vi "Data_get_joe_3.3.vi"() -> ()   [LabVIEW 2011]
uses:
  <vilib>/Utility/error.llb/DialogType.ctl
  <vilib>/Analysis/2dsp.llb/Real FFT.vi
  <vilib>/Analysis/NI_AALPro.lvlib
panel:
  out "Tab Control":T1(tab)
  in  "freq. step (GHz)":dbl=0.0003 min=0.00025 max=67.0 step=1e-06 format="%#.12f"
  in  "number of steps":u32=1 min=1 step=1
  in  "Filter up to (MHz)":ext=2.5
  in  "Chirp start (MHz)":ext=2.5
  in  "Channel Number":u16=1
  in  "Amount of averagings":u32=10 min=1 step=1
  out "Busy":bool
  out "#points":u32
  out "read time (ms)":u32
  in  "time/div":T2(ring)
  in  "time/point":T3(ring)
  in  "TDS VISA Port":refnum<visa-resource-name>="GPIB0::1::INSTR"
  in  "PSG1 VISA Port":refnum<visa-resource-name>="GPIB0::1::INSTR"
  in  "PSG1 start freq. (GHz)":dbl=0.0003 min=0.00025 max=67.0 step=1e-06 format="%#.12f"
  in  "PSG1 Ampl (dBm)":dbl min=-135.0 max=30.0 step=0.5 format="%#_8g"
  in  "Auto":bool caption="Autosave"
  in  "Automatic Overwrite?":bool
  out "f cur. (GHz)":i32
  in  "File Extension":string="ccd"
  in  "File Name":string="trace"
  in  "Folder":path
  in  "PSG2 Ampl (dBm)":dbl min=-135.0 max=30.0 step=0.5 format="%#_8g"
  in  "PSG2 freq. offset (GHz)":dbl=0.0003 min=0.00025 max=67.0 step=1e-06 format="%#.12f"
  in  "PSG2 VISA Port":refnum<visa-resource-name>="GPIB0::1::INSTR"
  in  "Chirp up to (GHz)":dbl
  in  "#Sweeps":u32=1 min=1 max=1000 step=1
  out "Current sweep":u32=1 min=1 max=1000 step=1
  in  "FFT every#":u32=1 min=1 max=1000 step=1
  in  "Substr":bool
  out "Frequency Domain Signal":cluster{ext[], dbl[]}(graph)
  out "Time Domain Signal":dbl[](graph)
  out "Data":dbl[](array[numeric])
  out "FFT (Im)":dbl[](array[numeric])
  out "FFT (Re)":dbl[](array[numeric])
  out "Final array":ext[][](array[numeric])
  out "size(s)":i32
  out "tdsavges#":i32 caption="tds averaged:"
  out "Oscilloscope Data":dbl[](array[numeric])
  in  "PauseB":bool caption="Pause"
  in  "Start":bool
  in  "Quit":bool
  in  "Stop":bool
  # "General Settings"
  # "OSC Settings"
  # "PSG1 Settings"
  # "PSG2 Settings"
  # "File Storage"
  # "Spectrum data"
  # "Vi Control"
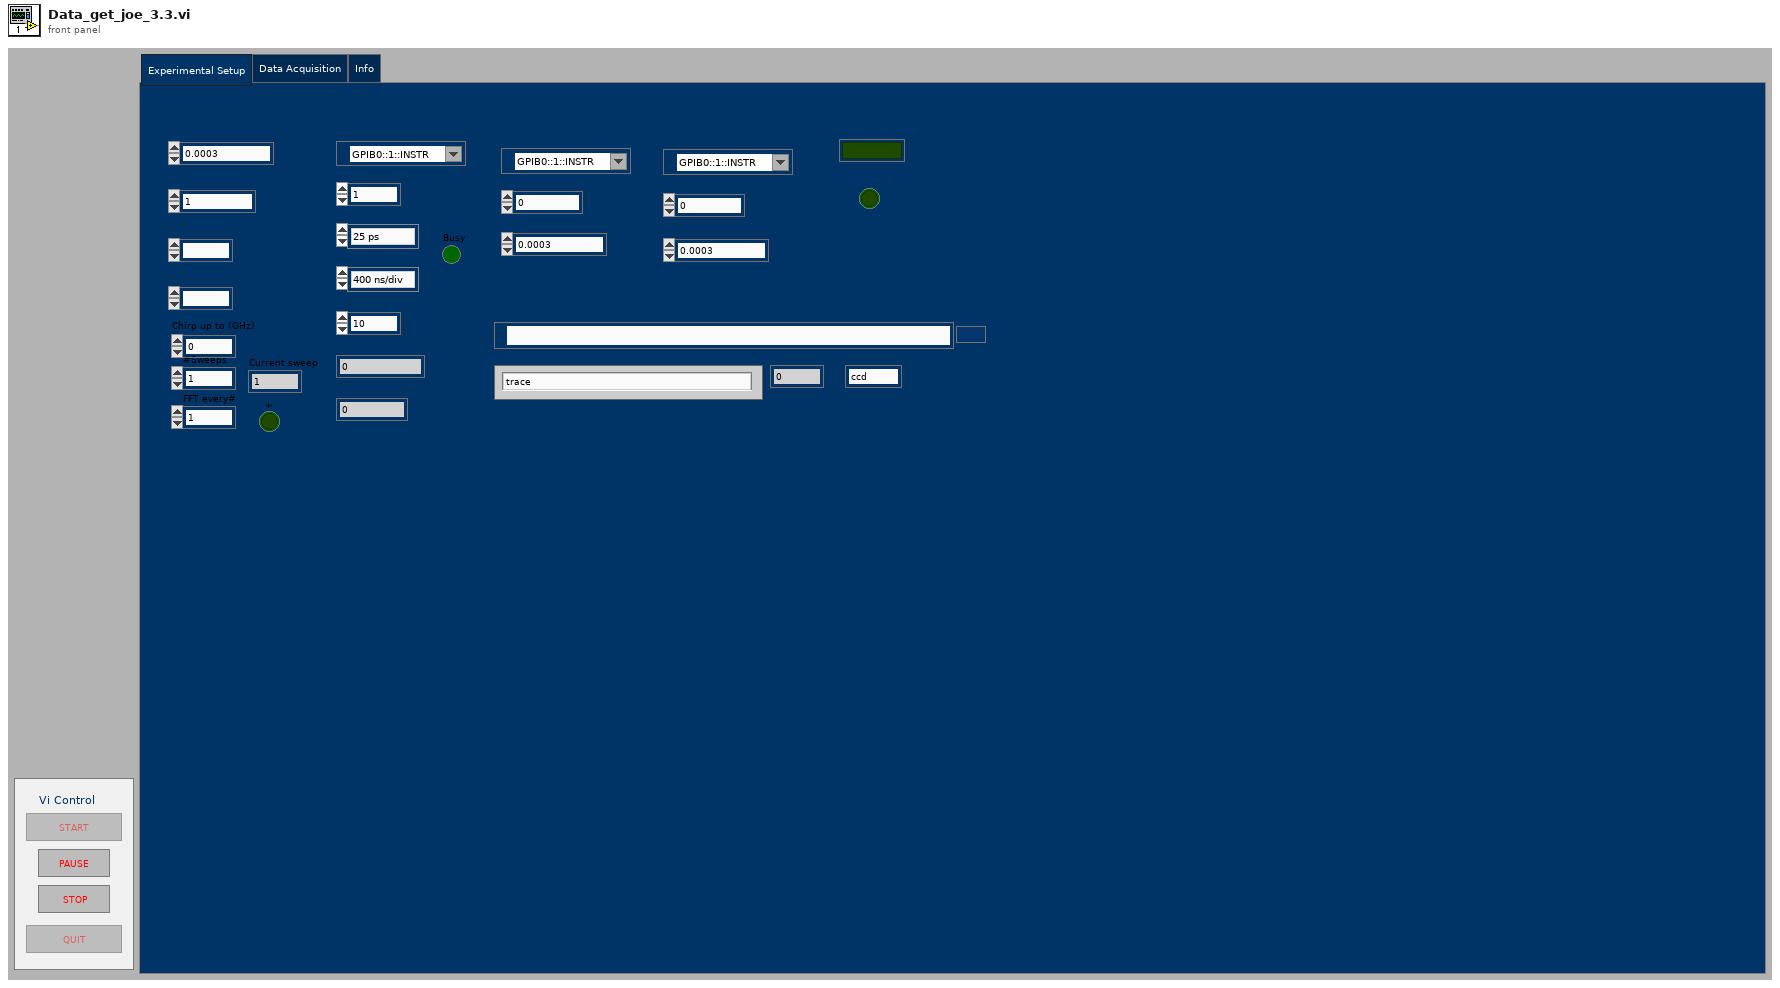
[diagram p1: front panel]
types:
  T1 = enum32{"Experimental Setup", "Data Acquisition", "Info"}
  T2 = enum16{"400 ns/div", "1 us/div", "2 us/div", "4 us/div", "10 us/div", "20 us/div"}
  T3 = enum16{"25 ps", "50 ps", "100 ps", "200 ps", "400 ps", "800 ps", "2 ns"}
  T4 = enum8{"Enabled", "Disabled", "Disabled and Grayed Out"}
  T5 = enum16{"open", "replace", "create", "open or create", "replace or create", "replace or create with confirmation"}
  T6 = typedef "DialogType.ctl" = u16
  T7 = cluster{"Folder":path, "File Name":string, "File Extension":string}
  T8 = cluster{"Folder":path, "Name":string, "Ext":string}
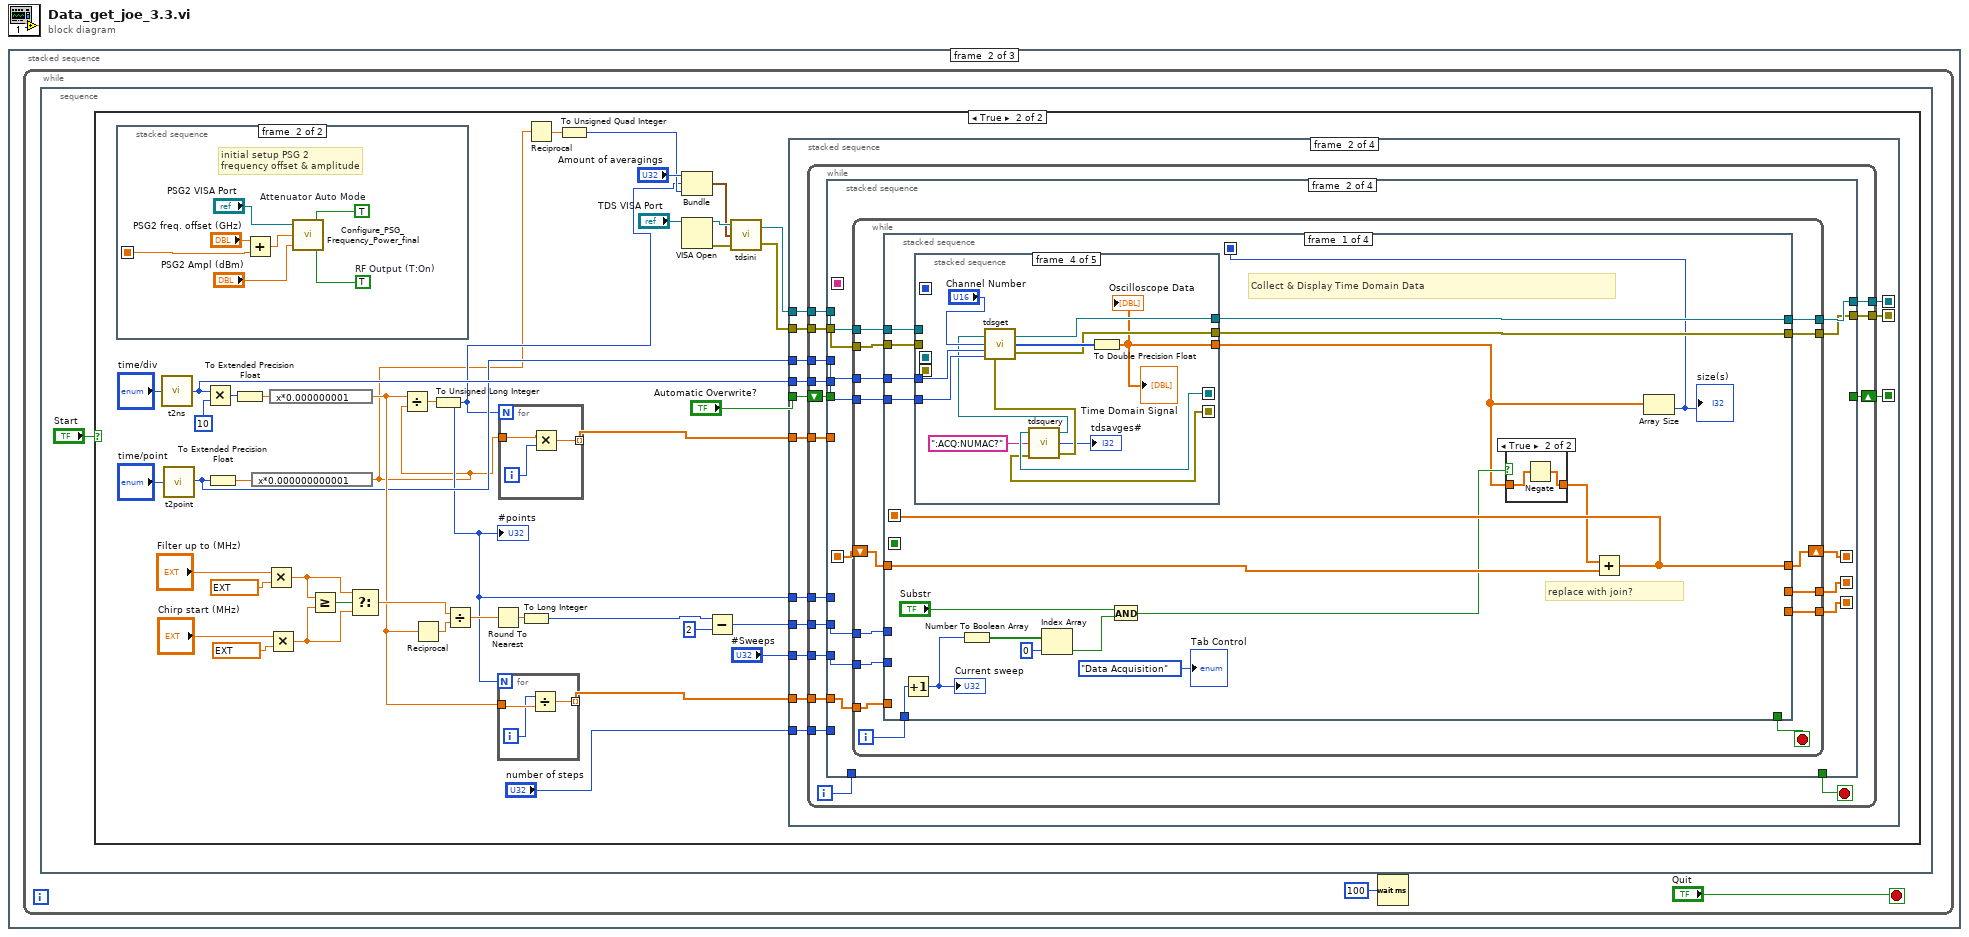
[diagram p0: block diagram]
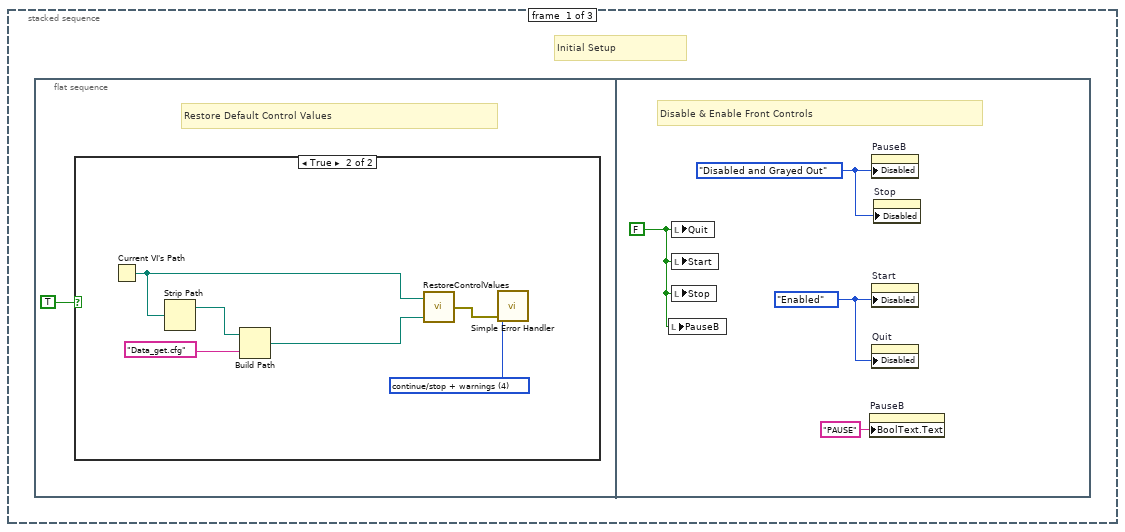
[diagram p2: hidden frame]
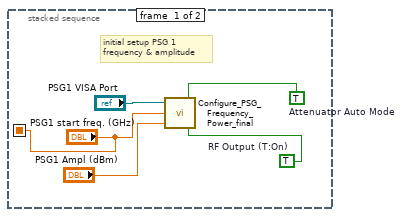
[diagram p5: hidden frame]
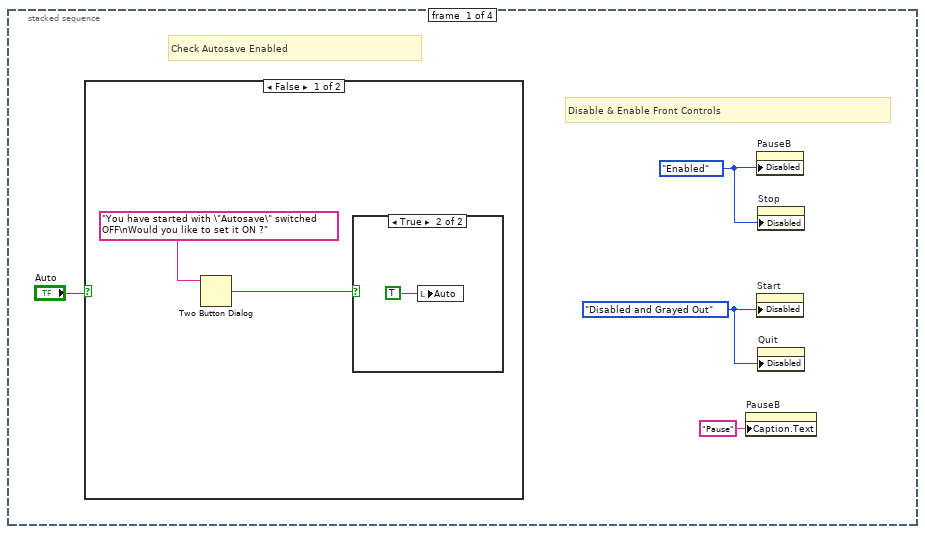
[diagram p6: hidden frame]
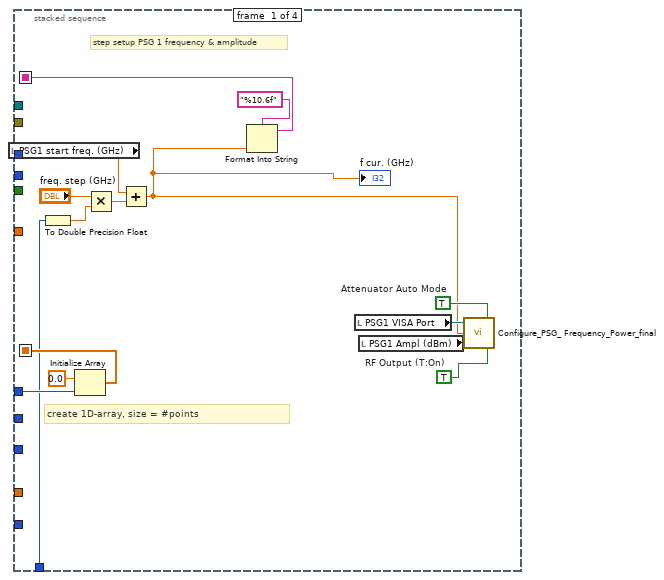
[diagram p9: hidden frame]
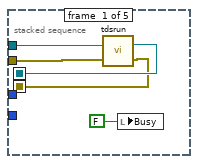
[diagram p11: hidden frame]
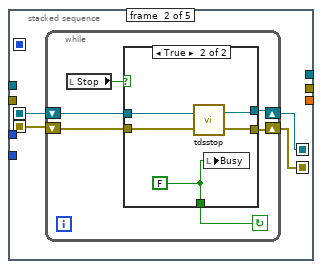
[diagram p12: hidden frame]
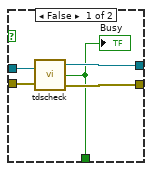
[diagram p13: hidden frame]
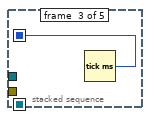
[diagram p14: hidden frame]
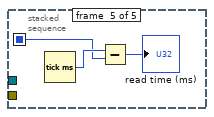
[diagram p15: hidden frame]
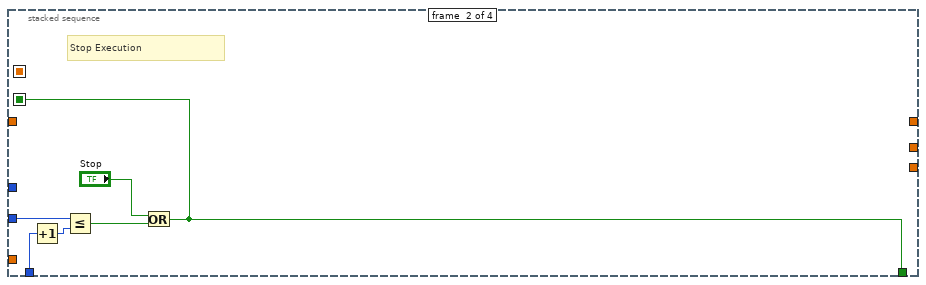
[diagram p16: hidden frame]
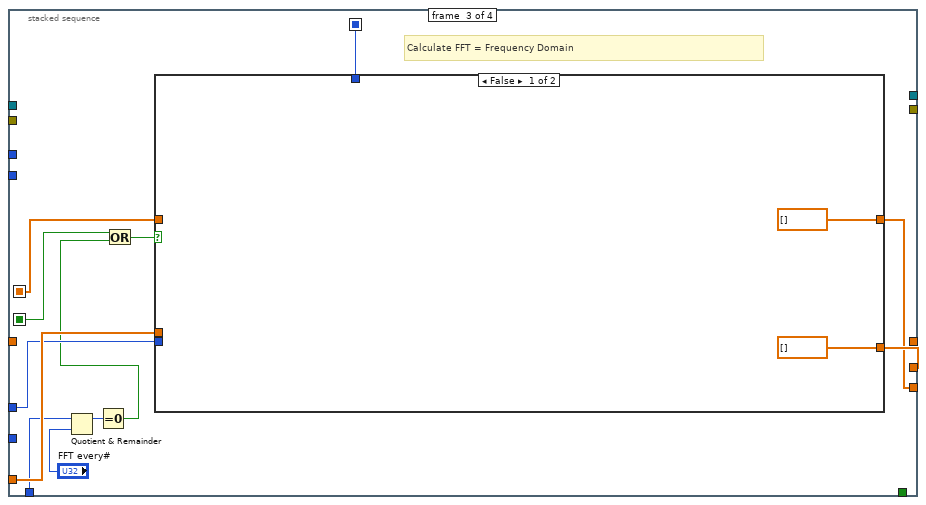
[diagram p17: hidden frame]
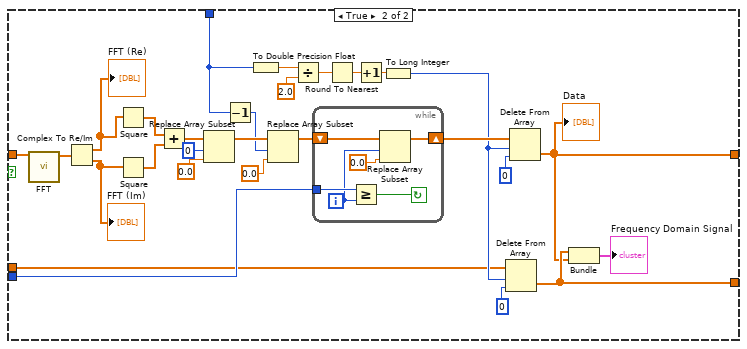
[diagram p18: hidden frame]
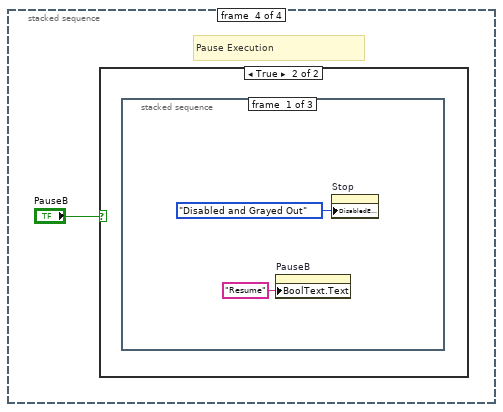
[diagram p19: hidden frame]
diagram:
  n1 = stacked-sequence {
    frame #0 {
      # "Initial Setup"
      n2 = flat-sequence {
        frame #0 {
          # "Restore Default Control Values"
          n3 = case shown="True" TRUE {
            frame False {
            }
            frame True {
              w2 = T6 4 items=["no dialog", "OK message", "continue or stop message", "OK message + warnings", "continue/stop + warnings"] ("type of dialog (OK msg:1)")
              n4 = Current VI's Path() -> (path=w3:path)
              n5 = Strip Path(path=w3) -> (stripped path=w4:path)  [unwired: 1 out]
              n6 = Build Path(base path=w4, name or relative path="Data_get.cfg") -> (appended path=w6:path)
              n7 = call "RestoreControlValues.vi"("file path"=w6, "vi path"=w3) -> ("error out"=w5:errorcluster)
              n8 = call <vilib>:"Simple Error Handler.vi"("type of dialog (OK msg:1)"=w2, "error in (no error)"=w5) -> ()  [unwired: 3 in, 5 out]
            }
          }
        }
        frame #1 {
          w10 = T4."Disabled and Grayed Out" ("Disabled")
          w8 = T4."Enabled" ("Disabled")
          w11 = FALSE ("Quit")
          # "Disable & Enable Front Controls"
          n9 = local write "PauseB"(w11) -> ()
          n10 = local write "Quit"(w11) -> ()
          n11 = local write "Start"(w11) -> ()
          n12 = local write "Stop"(w11) -> ()
          n13 = property on="PauseB" class="Bool (strict)"("BoolText.Text"="PAUSE" ("Boolean Text.Text")) -> ()  [unwired: 2 in, 2 out]
          n14 = property on="PauseB" class="Bool (strict)"("Disabled"=w10) -> ()  [unwired: 2 in, 2 out]
          n15 = property on="Start" class="Bool (strict)"("Disabled"=w8) -> ()  [unwired: 2 in, 2 out]
          n16 = property on="Quit" class="Bool (strict)"("Disabled"=w8) -> ()  [unwired: 2 in, 2 out]
          n17 = property on="Stop" class="Bool (strict)"("Disabled"=w10) -> ()  [unwired: 2 in, 2 out]
        }
      }
    }
    frame #1 {
      n18 = while {
        stop <- "Quit" stop-if-true
        n19 = stacked-sequence {
          frame #0 {
            n20 = case shown="True" "Start" {
              frame False {
              }
              frame True {
                n21 = stacked-sequence {
                  seq-local: ["PSG1 start freq. (GHz)" _] -> [_ w63]
                  frame #0 {
                    w59 = TRUE  # Attenuator Auto Mode
                    w57 = TRUE  # RF Output (T:On)
                    # "initial setup PSG 1 \nfrequency & amplitude"
                    n22 = call "Configure_PSG_ Frequency_Power_final.vi"("RF Output (T:On)"=w57, "Attenuator Auto Mode (T:Enable)"=w59, "Power [dBm]"="PSG1 Ampl (dBm)", "Frequency [GHz]"="PSG1 start freq. (GHz)", "VISA resource name"="PSG1 VISA Port") -> ()
                  }
                  frame #1 {
                    w65 = TRUE  # Attenuator Auto Mode
                    w66 = TRUE  # RF Output (T:On)
                    # "initial setup PSG 2\nfrequency offset & amplitude"
                    n23 = Add(x="PSG2 freq. offset (GHz)", y=w63) -> (x+y=w62:dbl)
                    n24 = call "Configure_PSG_ Frequency_Power_final.vi"("RF Output (T:On)"=w66, "Attenuator Auto Mode (T:Enable)"=w65, "Power [dBm]"="PSG2 Ampl (dBm)", "Frequency [GHz]"=w62, "VISA resource name"="PSG2 VISA Port") -> ()
                  }
                }
                n25 = call "t2ns.vi"("t/div"="time/div") -> ("ns/div"=w27:u32)
                n26 = call "t2point.vi"("t/point"="time/point") -> ("ps/point"=w25:u32)
                n27 = Multiply(x=w27, y=u32 10) -> (x*y=w49:u32)
                n28 = To Extended Precision Float(1:w25) -> (0:w46:ext)
                n29 = To Extended Precision Float(1:w49) -> (0:w47:ext)
                n30 = expression code="x*0.000000000001"(w46) -> (w15:ext)
                n31 = Multiply(x="Filter up to (MHz)", y=ext 1000000.0) -> (x*y=w38:ext)
                n32 = Multiply(x="Chirp start (MHz)", y=ext 1000000.0) -> (x*y=w35:ext)
                n33 = expression code="x*0.000000001"(w47) -> (w29:ext)
                n34 = Greater Or Equal?(x=w38, y=w35) -> (x >= y?=w45:bool)
                n35 = Select(t=w38, s=w45, f=w35) -> (s? t:f=w43:ext)
                n36 = Divide(x=w29, y=w15) -> (x/y=w48:ext)
                n37 = Reciprocal(x=w29) -> (1/x=w44:ext)
                n38 = To Unsigned Long Integer(number=w48) -> (unsigned 32bit integer=w16:u32)
                "#points" <- w16
                n39 = Divide(x=w43, y=w44) -> (x/y=w42:ext)
                n40 = Round To Nearest(number=w42) -> (nearest integer value=w41:ext)
                n41 = for {
                  N: w16 -> [_]
                  tunnel: w29 -> [w463]
                  tunnel: [w464] -> w30 mode=indexing
                  i -> [w462]
                  n42 = Divide(x=w462, y=w463) -> (x/y=w464:ext)
                }
                n43 = for {
                  N: w16 -> [_]
                  tunnel: w15 -> [w467]
                  tunnel: [w466] -> w28 mode=indexing
                  i -> [w465]
                  n44 = Multiply(x=w467, y=w465) -> (x*y=w466:ext)
                }
                n45 = To Long Integer(number=w41) -> (32bit integer=w21:i32)
                n46 = Reciprocal(x=w15) -> (1/x=w31:ext)
                n47 = To Unsigned Quad Integer(1:w31) -> (0:w32:u64)
                n48 = Bundle("Amount of averagings"="Amount of averagings", w16, w32) -> (w33:cluster{"Amount of averagings ":u32, u32, u64})  [unwired: 1 in]
                n49 = VISA Open(VISA resource name="TDS VISA Port") -> (VISA resource name=w51:refnum<visa-resource-name>, error out=w52:errorcluster)  [unwired: 4 in]
                n50 = Subtract(x=w21, y=2) -> (x-y=w19:i32)
                n51 = call "tdsini.vi"("Error In (No Error)"=w52, "Acq_par"=w33, "VISA Port In"=w51) -> ("Error Out"=w53:errorcluster, "VISA Port Out"=w54:refnum<visa-resource-name>)
                n52 = stacked-sequence {
                  seq-local: [_ w80 _ _] -> [_ _ w423 _]
                  seq-local: [_ w79 _ _] -> [_ _ w422 _]
                  seq-local: [_ w74 _ _] -> [_ _ _ w424]
                  tunnel: w54 -> [_ w87 _ _]
                  tunnel: w53 -> [_ w86 _ _]
                  tunnel: w25 -> [_ w85 _ _]
                  tunnel: w27 -> [_ w84 _ _]
                  tunnel: w19 -> [_ w83 _ _]
                  tunnel: w30 -> [_ w82 _ _]
                  tunnel: "#Sweeps" -> [_ w81 _ _]
                  tunnel: w28 -> [_ w76 _ _]
                  tunnel: w16 -> [_ w78 _ _]
                  tunnel: "number of steps" -> [_ w77 _ _]
                  tunnel: "Automatic Overwrite?" -> [_ w75 _ _]
                  frame #0 {
                    w68 = T4."Enabled" ("Disabled")
                    w67 = T4."Disabled and Grayed Out" ("Disabled")
                    # "Check Autosave Enabled"
                    # "Disable & Enable Front Controls"
                    n53 = case shown="False" "Auto" {
                      frame False {
                        n54 = Two Button Dialog(message="You have started with \"Autosave\" switched OFF\nWould you like to set it ON ?") -> (T button?=w71:bool)  [unwired: 2 in]
                        n55 = case shown="True" w71 {
                          frame False {
                          }
                          frame True {
                            n56 = local write "Auto"(TRUE) -> ()
                          }
                        }
                      }
                      frame True {
                      }
                    }
                    n57 = property on="PauseB" class="Bool (strict)"("Caption.Text"="Pause") -> ()  [unwired: 2 in, 2 out]
                    n58 = property on="PauseB" class="Bool (strict)"("Disabled"=w68) -> ()  [unwired: 2 in, 2 out]
                    n59 = property on="Start" class="Bool (strict)"("Disabled"=w67) -> ()  [unwired: 2 in, 2 out]
                    n60 = property on="Stop" class="Bool (strict)"("Disabled"=w68) -> ()  [unwired: 2 in, 2 out]
                    n61 = property on="Quit" class="Bool (strict)"("Disabled"=w67) -> ()  [unwired: 2 in, 2 out]
                  }
                  frame #1 {
                    n62 = while {
                      tunnel: w87 -> [w103]
                      tunnel: w86 -> [w102]
                      tunnel: w85 -> [w101]
                      tunnel: w84 -> [w100]
                      tunnel: w83 -> [w99]
                      tunnel: w82 -> [w98]
                      tunnel: w81 -> [w97]
                      tunnel: [w96] -> w80
                      tunnel: [w95] -> w79
                      tunnel: w78 -> [w94]
                      tunnel: w77 -> [w92]
                      tunnel: w76 -> [w90]
                      shift-right: [w88] -> w74
                      shift-left: w75 -> [w89]
                      i -> [w93]
                      stop <- w91 stop-if-true
                      n63 = stacked-sequence {
                        seq-local: [w117 _ _ _] -> [_ w122 _ _]
                        seq-local: [_ w121 _ _] -> [_ _ w278 _]
                        seq-local: [_ w120 _ _] -> [_ _ w277 _]
                        seq-local: [_ w119 _ _] -> [_ _ w276 _]
                        seq-local: [w109 _ _ _] -> [_ _ w275 _]
                        tunnel: w103 -> [_ w131 _ _]
                        tunnel: w102 -> [_ w130 _ _]
                        tunnel: w101 -> [_ w129 _ _]
                        tunnel: w100 -> [_ w128 _ _]
                        tunnel: w99 -> [_ w127 _ _]
                        tunnel: w98 -> [_ w126 _ _]
                        tunnel: w97 -> [_ w125 _ _]
                        tunnel: [_ w124 _ _] -> w96
                        tunnel: [_ w123 _ _] -> w95
                        tunnel: w94 -> [w116 _ _ _]
                        tunnel: w93 -> [w113 _ _ w416]
                        tunnel: w92 -> [_ _ _ w415]
                        tunnel: [_ _ _ w414] -> w91
                        tunnel: w90 -> [_ _ w279 _]
                        tunnel: w89 -> [_ _ w273 _]
                        tunnel: [_ _ w272 _] -> w88
                        frame #0 {
                          w108 = TRUE  # Attenuator Auto Mode
                          w107 = TRUE  # RF Output (T:On)
                          # "step setup PSG 1 frequency & amplitude"
                          # "create 1D-array, size = #points"
                          n64 = local read "PSG1 start freq. (GHz)"() -> (w111:dbl)
                          n65 = To Double Precision Float(number=w113) -> (double precision float=w114:dbl)
                          n66 = Initialize Array(0.0 ("element"), w116) -> (w117:dbl[])
                          n67 = Multiply(x="freq. step (GHz)", y=w114) -> (x*y=w112:dbl)
                          n68 = Add(x=w111, y=w112) -> (x+y=w105:dbl)
                          "f cur. (GHz)" <- w105
                          n69 = Format Into String(format string="%10.6f", w105) -> (resulting string=w109:string)  [unwired: 2 in, 1 out]
                          n70 = local read "PSG1 VISA Port"() -> (w106:refnum<visa-resource-name>)
                          n71 = local read "PSG1 Ampl (dBm)"() -> (w104:dbl)
                          n72 = call "Configure_PSG_ Frequency_Power_final.vi"("RF Output (T:On)"=w107, "Attenuator Auto Mode (T:Enable)"=w108, "Power [dBm]"=w104, "Frequency [GHz]"=w105, "VISA resource name"=w106) -> ()
                        }
                        frame #1 {
                          n73 = while {
                            tunnel: [w143] -> w123
                            tunnel: [w144] -> w124
                            tunnel: w130 -> [w145]
                            tunnel: w131 -> [w146]
                            tunnel: w129 -> [w142]
                            tunnel: w128 -> [w141]
                            tunnel: w126 -> [w139]
                            tunnel: w127 -> [w140]
                            tunnel: w125 -> [w136]
                            shift-right: [w134] -> w121
                            shift-left: w122 -> [w135]
                            tunnel: [w133] -> w120
                            tunnel: [w132] -> w119
                            i -> [w138]
                            stop <- w137 stop-if-true
                            n74 = stacked-sequence {
                              seq-local: [w158 _ _ _] -> [_ _ w228 _]
                              seq-local: [w159 _ _ _] -> [_ _ w227 _]
                              seq-local: [_ w211 _ _] -> [_ _ w218 _]
                              tunnel: w146 -> [w165 _ _ _]
                              tunnel: w145 -> [w148 _ _ _]
                              tunnel: [w164 _ _ _] -> w144
                              tunnel: [w163 _ _ _] -> w143
                              tunnel: w142 -> [w162 _ _ _]
                              tunnel: w141 -> [w161 _ _ _]
                              tunnel: w140 -> [_ _ w225 _]
                              tunnel: w139 -> [_ _ w226 _]
                              tunnel: w138 -> [w157 w216 w222 _]
                              tunnel: [_ w211 _ _] -> w137
                              tunnel: w136 -> [_ w213 _ _]
                              tunnel: w135 -> [w160 _ _ _]
                              tunnel: [w159 _ _ _] -> w134
                              tunnel: [_ _ w224 _] -> w133
                              tunnel: [_ _ w223 _] -> w132
                              frame #0 {
                                # "replace with join?"
                                # "Collect & Display Time Domain Data"
                                n75 = Increment(x=w157) -> (x+1=w149:i32)
                                "Current sweep" <- w149
                                n76 = stacked-sequence {
                                seq-local: [w171 _ _ _ _] -> [_ w177 _ _ _]
                                seq-local: [w170 _ _ _ _] -> [_ w176 _ _ _]
                                seq-local: [_ w174 _ _ _] -> [_ _ _ w199 _]
                                seq-local: [_ w175 _ _ _] -> [_ _ _ w200 _]
                                seq-local: [_ _ w194 _ _] -> [_ _ _ _ w209]
                                tunnel: w165 -> [w172 _ _ _ _]
                                tunnel: w148 -> [w173 _ _ _ _]
                                tunnel: [_ _ _ w206 _] -> w164
                                tunnel: [_ _ _ w205 _] -> w163
                                tunnel: w162 -> [_ _ _ w203 _]
                                tunnel: w161 -> [_ _ _ w202 _]
                                tunnel: [_ _ _ w201 _] -> w152
                                frame #0 {
                                n77 = call "tdsrun.vi"("Error In (No Error)"=w173, "VISA Port In"=w172) -> ("Error Out"=w170:errorcluster, "VISA Port Out"=w171:refnum<visa-resource-name>)
                                n78 = local write "Busy"(FALSE ("Busy")) -> ()
                                }
                                frame #1 {
                                n79 = while {
                                shift-right: [w181] -> w175
                                shift-left: w177 -> [w182]
                                shift-right: [w180] -> w174
                                shift-left: w176 -> [w183]
                                stop <- w179 continue-if-true
                                n80 = local read "Stop"() -> (w178:bool)
                                n81 = case shown="True" w178 {
                                tunnel: w183 -> [w188 w192]
                                tunnel: w182 -> [w187 w193]
                                tunnel: [w186 w190] -> w181
                                tunnel: [w185 w191] -> w180
                                tunnel: [w184 w189] -> w179
                                frame False {
                                n82 = call "tdscheck.vi"("VISA Port In"=w187, "Error In (No Error)"=w188) -> ("VISA Port Out"=w186:refnum<visa-resource-name>, "busy"=w184:bool, "Error Out"=w185:errorcluster)
                                "Busy" <- w184
                                }
                                frame True {
                                w189 = FALSE ("busy")
                                n83 = call "tdsstop.vi"("Error In (No Error)"=w192, "VISA Port In"=w193) -> ("Error Out"=w191:errorcluster, "VISA Port Out"=w190:refnum<visa-resource-name>)
                                n84 = local write "Busy"(w189) -> ()
                                }
                                }
                                }
                                }
                                frame #2 {
                                n85 = Tick Count (ms)() -> (millisecond timer value=w194:u32)
                                }
                                frame #3 {
                                n86 = call "tdsquery.vi"("Error In (No Error)"=w199, "String to TDS"=":ACQ:NUMAC?", "VISA Port In"=w200) -> ("Error Out"=w196:errorcluster, "number"=→"tdsavges#":i32, "VISA Port Out"=w197:refnum<visa-resource-name>)
                                n87 = call "tdsget.vi"("VISA Port In"=w197, "Channel Number"="Channel Number", "ps/point"=w203, "ns/div"=w202, "Error In (No Error)"=w196) -> ("VISA Port Out"=w206:refnum<visa-resource-name>, "TDS Data"=w207:u16[], "Error Out"=w205:errorcluster)  [unwired: 8 in]
                                n88 = To Double Precision Float(number=w207) -> (double precision float=w201:dbl[])
                                "Time Domain Signal" <- w201
                                "Oscilloscope Data" <- w201
                                }
                                frame #4 {
                                n89 = Tick Count (ms)() -> (millisecond timer value=w210:u32)
                                n90 = Subtract(x=w210, y=w209) -> (x-y=→"read time (ms)":u32)
                                }
                                }
                                n91 = Number To Boolean Array(number=w149) -> (Boolean array=w156:bool[])
                                n92 = Index Array(array=w156, index=0) -> (element=w154:bool)
                                n93 = And(x="Substr", y=w154) -> (x .and. y?=w153:bool)
                                n94 = case shown="True" w153 {
                                tunnel: w152 -> [w166 w168]
                                tunnel: [w166 w167] -> w151
                                frame False {
                                }
                                frame True {
                                n95 = Negate(x=w168) -> (-x=w167:dbl[])
                                }
                                }
                                n96 = Add(x=w151, y=w160) -> (x+y=w159:dbl[])
                                n97 = Array Size(array=w152) -> (size(s)=w158:i32)
                                "size(s)" <- w158
                                "Tab Control" <- T1."Data Acquisition" ("Tab Control")
                              }
                              frame #1 {
                                # "Stop Execution"
                                n98 = Increment(x=w216) -> (x+1=w212:i32)
                                n99 = Less Or Equal?(x=w213, y=w212) -> (x <= y?=w215:bool)
                                n100 = Or(x="Stop", y=w215) -> (x .or. y?=w211:bool)
                              }
                              frame #2 {
                                # "Calculate FFT = Frequency Domain"
                                n101 = Quotient & Remainder(x=w222, y="FFT every#") -> (x-y*floor(x/y)=w220:u32)  [unwired: 1 out]
                                n102 = Equal To 0?(x=w220) -> (x = 0?=w217:bool)
                                n103 = Or(x=w218, y=w217) -> (x .or. y?=w219:bool)
                                n104 = case shown="False" w219 {
                                tunnel: w228 -> [_ w236]
                                tunnel: w227 -> [_ w235]
                                tunnel: w226 -> [_ w231]
                                tunnel: w225 -> [_ w234]
                                tunnel: [ext[] [] w233] -> w224
                                tunnel: [dbl[] [] w232] -> w223
                                frame False {
                                }
                                frame True {
                                n105 = call-poly <vilib>:"FFT.vi"("X"=w235) -> ("FFT {X}"=w258:cdb[])  [unwired: 9 in, 1 out]
                                n106 = Complex To Re/Im(x + iy=w258) -> (x=w257:dbl[], y=w256:dbl[])
                                "FFT (Re)" <- w257
                                "FFT (Im)" <- w256
                                n107 = Square(x=w257) -> (x^2=w255:dbl[])
                                n108 = Square(x=w256) -> (x^2=w254:dbl[])
                                n109 = Add(x=w255, y=w254) -> (x+y=w250:dbl[])
                                n110 = Replace Array Subset(array=w250, new element=0.0 ("new element/subarray"), index=0) -> (w249:dbl[])
                                n111 = Decrement(x=w236) -> (x-1=w248:i32)
                                n112 = To Double Precision Float(number=w236) -> (double precision float=w244:dbl)
                                n113 = Replace Array Subset(array=w249, new element=0.0 ("new element/subarray"), index=w248) -> (w246:dbl[])
                                n114 = Divide(x=w244, y=2.0) -> (x/y=w242:dbl)
                                n115 = while {
                                tunnel: w234 -> [w263]
                                shift-right: [w261] -> w245
                                shift-left: w246 -> [w262]
                                i -> [w260]
                                stop <- w264 continue-if-true
                                n116 = Greater Or Equal?(x=w263, y=w260) -> (x >= y?=w264:bool)
                                n117 = Replace Array Subset(array=w262, new element=0.0 ("new element/subarray"), index=w260) -> (w261:dbl[])
                                }
                                n118 = Round To Nearest(number=w242) -> (nearest integer value=w241:dbl)
                                n119 = Increment(x=w241) -> (x+1=w240:dbl)
                                n120 = To Long Integer(number=w240) -> (32bit integer=w237:i32)
                                n121 = Delete From Array(array=w231, length=w237, index=0) -> (deleted portion=w233:ext[])  [unwired: 1 out]
                                n122 = Delete From Array(array=w245, length=w237, index=0) -> (deleted portion=w232:dbl[])  [unwired: 1 out]
                                "Data" <- w232
                                n123 = Bundle(w233, w232) -> (→"Frequency Domain Signal":cluster{ext[], dbl[]})  [unwired: 1 in]
                                }
                                }
                              }
                              frame #3 {
                                # "Pause Execution"
                                n124 = case shown="True" "PauseB" {
                                frame False {
                                }
                                frame True {
                                n125 = stacked-sequence {
                                frame #0 {
                                n126 = property on="PauseB" class="Bool (strict)"("BoolText.Text"="Resume" ("Caption.Text")) -> ()  [unwired: 2 in, 2 out]
                                n127 = property on="Stop" class="Bool (strict)"("DisabledEnum"=T4."Disabled and Grayed Out" ("Disabled")) -> ()  [unwired: 2 in, 2 out]
                                }
                                frame #1 {
                                n128 = while {
                                stop <- w269 continue-if-true
                                n129 = local read "PauseB"() -> (w269:bool)
                                n130 = Wait Until Next ms Multiple(millisecond multiple=u32 150) -> ()  [unwired: 1 out]
                                }
                                }
                                frame #2 {
                                n131 = property on="PauseB" class="Bool (strict)"("BoolText.Text"="Pause" ("Caption.Text")) -> ()  [unwired: 2 in, 2 out]
                                n132 = property on="Stop" class="Bool (strict)"("DisabledEnum"=T4."Enabled" ("Disabled")) -> ()  [unwired: 2 in, 2 out]
                                }
                                }
                                }
                                }
                              }
                            }
                          }
                        }
                        frame #2 {
                          # "Auto Safe?"
                          n133 = local read "Auto"() -> (w274:bool)
                          n134 = case shown="True" w274 {
                            tunnel: w279 -> [_ w287]
                            tunnel: w278 -> [_ w286]
                            tunnel: w277 -> [_ w285]
                            tunnel: w276 -> [_ w284]
                            tunnel: w275 -> [_ w283]
                            tunnel: w273 -> [_ w282]
                            tunnel: [FALSE w281] -> w272
                            frame False {
                            }
                            frame True {
                              n135 = stacked-sequence {
                                seq-local: [w288 _ _ _] -> [_ w312 _ _]
                                seq-local: [_ _ w366 _] -> [_ _ _ w406]
                                seq-local: [_ w298 _ _] -> [_ _ _ w397]
                                tunnel: w287 -> [_ w314 _ _]
                                tunnel: w286 -> [_ w301 _ _]
                                tunnel: w285 -> [_ _ _ w409]
                                tunnel: w284 -> [_ _ _ w408]
                                tunnel: w283 -> [w291 w300 w368 _]
                                tunnel: w282 -> [_ w304 _ _]
                                tunnel: [_ w298 _ _] -> w281
                                frame #0 {
                                # "create complete filename incl. path as a string"
                                n136 = Path To String(path="Folder") -> (string=w296:string)
                                n137 = Concatenate Strings(w296, "\\\\" ("string"), "File Name", "_", "td", w291, ".", "File Extension") -> (w288:string)
                                }
                                frame #1 {
                                # "(%e) = Scientific Notation"
                                n138 = Build Array(w314, w301) -> (w316:ext[][])
                                n139 = String To Path(string=w312) -> (path=w303:path)
                                n140 = case shown="False" w304 {
                                tunnel: w312 -> [w318 _]
                                tunnel: [w323 w364] -> w298
                                tunnel: [w321 T5."replace or create" ("operation (0:open)")] -> w306
                                tunnel: w304 -> [w322 w364]
                                tunnel: w303 -> [w320 w363]
                                tunnel: [w319 w363] -> w302
                                tunnel: w300 -> [w317 _]
                                frame False {
                                n141 = call "CheckFileExist.vi"("Path"=w318) -> ("File Exists"=w325:bool, "Overwrite File"=w324:bool)  [unwired: 1 in, 1 out]
                                n142 = case "check file existance" shown="True" w325 {
                                tunnel: w324 -> [_ w334]
                                tunnel: [w328 w332] -> w323
                                tunnel: w322 -> [w328 _]
                                tunnel: [T5."create" ("operation (0:open)") w333] -> w321
                                tunnel: w320 -> [w326 w331]
                                tunnel: [w326 w330] -> w319
                                tunnel: w317 -> [_ w329]
                                frame False {
                                # "file doesn't exist"
                                }
                                frame True {
                                # "file exists"
                                n143 = case shown="False" w334 {
                                tunnel: [w337 T5."replace or create" ("operation (0:open)")] -> w333
                                tunnel: [w338 TRUE] -> w332
                                tunnel: w331 -> [_ w360]
                                tunnel: [w335 w360] -> w330
                                tunnel: w329 -> [w336 _]
                                frame False {
                                # "file exists and should not be overwritten"
                                n144 = stacked-sequence {
                                tunnel: [_ _ FALSE] -> w338
                                tunnel: [_ _ T5."create" ("operation (0:open)")] -> w337
                                tunnel: w336 -> [_ w347 _]
                                tunnel: [_ w352 _] -> w335
                                frame #0 {
                                # "enter new file name"
                                n145 = local read "File Extension"() -> (w344:string)
                                n146 = local read "File Name"() -> (w345:string)
                                n147 = local read "Folder"() -> (w346:path)
                                n148 = Bundle("Folder"=w346, "File Name"=w345, "File Extension"=w344) -> (w343:T7)  [unwired: 1 in]
                                n149 = call "ChangeFileName.vi"("input par"=w343) -> ("output par"=w342:T8)  [unwired: 1 out]
                                n150 = Unbundle(w342) -> ("Folder"=w341:path, "Name"=w340:string, "Ext"=w339:string)
                                n151 = local write "File Extension"(w339) -> ()
                                n152 = local write "File Name"(w340) -> ()
                                n153 = local write "Folder"(w341) -> ()
                                }
                                frame #1 {
                                # "create new path"
                                n154 = local read "File Extension"() -> (w349:string)
                                n155 = local read "File Name"() -> (w353:string)
                                n156 = local read "Folder"() -> (w354:path)
                                n157 = Path To String(path=w354) -> (string=w357:string)
                                n158 = Concatenate Strings(w357, "\\\\" ("string"), w353, "_", "td", w347, ".", w349) -> (w348:string)
                                n159 = String To Path(string=w348) -> (path=w352:path)
                                }
                                frame #2 {
                                }
                                }
                                }
                                frame True {
                                # "overwrite existing file"
                                }
                                }
                                }
                                }
                                }
                                frame True {
                                }
                                }
                                n160 = Transpose 2D Array(2D array=w316) -> (transposed array=w313:ext[][])
                                n161 = Array To Spreadsheet String(array=w313, 3:"%e") -> (spreadsheet string=w305:string)  [unwired: 1 in]
                                n162 = Open/Create/Replace File(file path (use dialog)=w302, operation (0:open)=w306, access (0:read/write)=enum16{"read/write", "read-only", "write-only"}."write-only") -> (refnum out=w308:refnum<file>, error out=w311:errorcluster)  [unwired: 3 in, 1 out]
                                n163 = Write to Text File(file (use dialog)=w308, text=w305, error in=w311) -> (refnum out=w309:refnum<file>, error out=w310:errorcluster)  [unwired: 1 in, 1 out]
                                n164 = Close File(refnum=w309, error in=w310) -> (error out=w299:errorcluster)  [unwired: 1 out]
                                n165 = call <vilib>:"Simple Error Handler.vi"("error in (no error)"=w299) -> ()  [unwired: 4 in, 5 out]
                                }
                                frame #2 {
                                n166 = local read "File Extension"() -> (w367:string)
                                n167 = local read "File Name"() -> (w369:string)
                                n168 = local read "Folder"() -> (w370:path)
                                n169 = Path To String(path=w370) -> (string=w376:string)
                                n170 = Concatenate Strings(w376, "\\\\" ("string"), w369, "_") -> (w371:string)
                                n171 = Concatenate Strings(w371, "sd", w368, ".", w367) -> (w366:string)
                                }
                                frame #3 {
                                n172 = Multiply(x="Chirp up to (GHz)", y=1000000000.0) -> (x*y=w378:dbl)
                                n173 = To Extended Precision Float(1:w378) -> (0:w377:ext)
                                n174 = To Extended Precision Float(1:w408) -> (0:w410:ext[])
                                n175 = Build Array(w409, w410) -> (w407:ext[][])
                                n176 = String To Path(string=w406) -> (path=w399:path)
                                n177 = case shown="True" w397 {
                                tunnel: [T5."replace or create with confirmation" ("operation (0:open)") T5."replace or create" ("operation (0:open)")] -> w398
                                frame False {
                                }
                                frame True {
                                }
                                }
                                n178 = Transpose 2D Array(2D array=w407) -> (transposed array=w380:ext[][])
                                n179 = Index Array(array=w380, index (col)=0 ("disabled index (col)")) -> (element=w390:ext[])  [unwired: 1 in]
                                n180 = Index Array(array=w390, index=1) -> (element=w392:ext)
                                n181 = Index Array(array=w390, index=0) -> (element=w391:ext)
                                n182 = Subtract(x=w392, y=w391) -> (x-y=w387:ext)
                                n183 = Divide(x=w377, y=w387) -> (x/y=w384:ext)
                                n184 = Round To Nearest(number=w384) -> (nearest integer value=w386:ext)
                                n185 = To Long Integer(number=w386) -> (32bit integer=w385:i32)
                                n186 = Increment(x=w385) -> (x+1=w381:i32)
                                n187 = Array Subset(array=w380, index (row)=0 ("index"), length (row)=w381, index (col)=0 ("index"), length (col)=w381) -> (w379:ext[][])
                                "Final array" <- w379
                                n188 = Array To Spreadsheet String(array=w379, 3:"%e") -> (spreadsheet string=w400:string)  [unwired: 1 in]
                                n189 = Open/Create/Replace File(file path (use dialog)=w399, operation (0:open)=w398, access (0:read/write)=enum16{"read/write", "read-only", "write-only"}."write-only") -> (refnum out=w402:refnum<file>, error out=w405:errorcluster)  [unwired: 3 in, 1 out]
                                n190 = Write to Text File(file (use dialog)=w402, text=w400, error in=w405) -> (refnum out=w403:refnum<file>, error out=w404:errorcluster)  [unwired: 1 in, 1 out]
                                n191 = Close File(refnum=w403, error in=w404) -> (error out=w396:errorcluster)  [unwired: 1 out]
                                n192 = call <vilib>:"Simple Error Handler.vi"("error in (no error)"=w396) -> ()  [unwired: 4 in, 5 out]
                                }
                              }
                            }
                          }
                        }
                        frame #3 {
                          n193 = Increment(x=w416) -> (x+1=w418:i32)
                          n194 = Less Or Equal?(x=w415, y=w418) -> (x <= y?=w419:bool)
                          n195 = local read "Stop"() -> (w417:bool)
                          n196 = Or(x=w417, y=w419) -> (x .or. y?=w414:bool)
                        }
                      }
                    }
                  }
                  frame #2 {
                    w421 = T4."Disabled and Grayed Out" ("Disabled")
                    w420 = T4."Enabled" ("Disabled")
                    n197 = property on="Quit" class="Bool (strict)"("Disabled"=w420) -> ()  [unwired: 2 in, 2 out]
                    n198 = property on="PauseB" class="Bool (strict)"("Disabled"=w421) -> ()  [unwired: 2 in, 2 out]
                    n199 = property on="Stop" class="Bool (strict)"("Disabled"=w421) -> ()  [unwired: 2 in, 2 out]
                    n200 = property on="Start" class="Bool (strict)"("Disabled"=w420) -> ()  [unwired: 2 in, 2 out]
                    n201 = VISA Close(VISA resource name=w423, error in (no error)=w422) -> ()  [unwired: 1 out]
                  }
                  frame #3 {
                    n202 = local read "Auto"() -> (w425:bool)
                    n203 = case shown="True" w425 {
                      tunnel: w424 -> [_ w428]
                      frame False {
                      }
                      frame True {
                        # "safe measurement settings to file"
                        n204 = local read "PSG1 start freq. (GHz)"() -> (w448:dbl)
                        n205 = local read "number of steps"() -> (w446:u32)
                        n206 = local read "PSG1 Ampl (dBm)"() -> (w451:dbl)
                        n207 = local read "freq. step (GHz)"() -> (w447:dbl)
                        n208 = local read "time/point"() -> (w457:T3)
                        n209 = local read "time/div"() -> (w456:T2)
                        n210 = local read "Channel Number"() -> (w458:u16)
                        n211 = local read "Amount of averagings"() -> (w455:u32)
                        n212 = local read "#Sweeps"() -> (w454:u32)
                        n213 = local read "Filter up to (MHz)"() -> (w453:ext)
                        n214 = local read "Chirp start (MHz)"() -> (w452:ext)
                        n215 = call "t2point.vi"("t/point"=w457) -> ("ps/point"=w449:u32)
                        n216 = call "t2ns.vi"("t/div"=w456) -> ("ns/div"=w450:u32)
                        n217 = local read "File Extension"() -> (w438:string)
                        n218 = local read "File Name"() -> (w441:string)
                        n219 = local read "Folder"() -> (w442:path)
                        n220 = Path To String(path=w442) -> (string=w445:string)
                        n221 = Format Into String(format string="Channel: %d\\nps/point: %d\\nns/div: %d\\nAmount of averagings: %d\\n#Sweeps: %d\\nFilter up to (MHz): %f\\nChirp start (MHz): %f\\nAmpl. (dBm): %f\\nf start (GHz): %f\\nf step (MHz): %f\\n#steps: %d\\n", w458, w449, w450, w455, w454, w453, w452, w451, w448, w447, w446) -> (resulting string=w429:string)  [unwired: 2 in, 1 out]
                        n222 = case shown="True" w428 {
                          tunnel: [T5."replace or create with confirmation" ("operation (0:open)") T5."replace or create" ("operation (0:open)")] -> w427
                          frame False {
                          }
                          frame True {
                          }
                        }
                        n223 = Concatenate Strings(w445, "\\\\" ("string"), w441, "_", "par", ".", w438) -> (w437:string)
                        n224 = String To Path(string=w437) -> (path=w431:path)
                        n225 = Open/Create/Replace File(file path (use dialog)=w431, operation (0:open)=w427, access (0:read/write)=enum16{"read/write", "read-only", "write-only"}."write-only") -> (refnum out=w433:refnum<file>, error out=w436:errorcluster)  [unwired: 3 in, 1 out]
                        n226 = Write to Text File(file (use dialog)=w433, text=w429, error in=w436) -> (refnum out=w434:refnum<file>, error out=w435:errorcluster)  [unwired: 1 in, 1 out]
                        n227 = Close File(refnum=w434, error in=w435) -> (error out=w432:errorcluster)  [unwired: 1 out]
                        n228 = call <vilib>:"Simple Error Handler.vi"("error in (no error)"=w432) -> ()  [unwired: 4 in, 5 out]
                      }
                    }
                    n229 = local write "Stop"(FALSE ("Stop")) -> ()
                  }
                }
              }
            }
          }
        }
        n230 = Wait (ms)(milliseconds to wait=u32 100) -> ()  [unwired: 1 out]
      }
    }
    frame #2 {
      n231 = Current VI's Path() -> (path=w468:path)
      n232 = Strip Path(path=w468) -> (stripped path=w469:path)  [unwired: 1 out]
      n233 = Build Path(base path=w469, name or relative path="Data_get.cfg") -> (appended path=w471:path)
      n234 = call "SaveControlValues.vi"("file path"=w471, "vi path"=w468) -> ("error out"=w470:errorcluster)
      n235 = call <vilib>:"Simple Error Handler.vi"("error in (no error)"=w470) -> ()  [unwired: 4 in, 5 out]
    }
  }
